vi "EX_REPORTS.vi"   [LabVIEW 2017]
uses:
  <vilib>/Utility/NIReport.llb/Append Report Text (str wrap).vi
  <vilib>/Utility/NIReport.llb/NI_report.lvclass
types:
  T1 = enum16{"maximized", "minimized", "normal", "no change"}
  T2 = cluster{"position (excel)":cluster{"row":i32, "column":i32}, "name (excel)":string, "bookmark (word)":string}
  T3 = enum16{"Standard Report", "HTML", "Word", "Excel"}
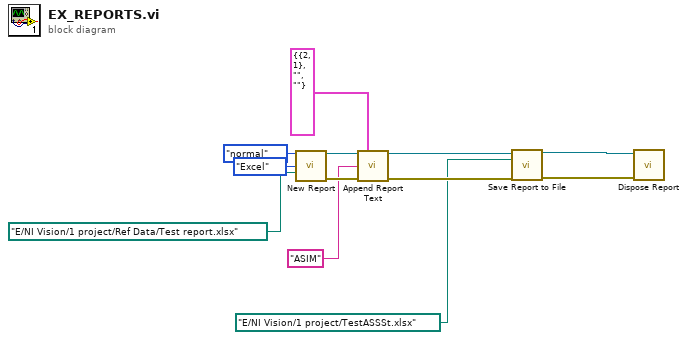
[diagram p0: block diagram]
diagram:
  n1 = call <vilib>:"New Report.vi"("window state (normal)"=T1."normal", "report type"=T3."Excel", "template (empty)"=path "E:/NI Vision/1 project/Ref Data/Test report.xlsx") -> ("report out"=w10:refnum<class "NI_report.lvclass">, "error out"=w9:errorcluster)  [unwired: 11 in]
  n2 = call-poly <vilib>:"Append Report Text.vi"("report in"=w10, "MS Office parameters"=T2 {"position (excel)"={"row"=2, "column"=1}, "name (excel)"="", "bookmark (word)"=""}, "text"="ASIM", "error in (no error)"=w9) -> ("report out"=w4:refnum<class "NI_report.lvclass">, "error out"=w6:errorcluster)  [unwired: 8 in, 2 out]
  n3 = call-dynamic "Save Report to File.vi"("report in"=w4, "report file path"=path "E:/NI Vision/1 project/TestASSSt.xlsx" ("template (empty)"), "error in (no error)"=w6) -> ("report out"=w3:refnum<class "NI_report.lvclass">, "error out"=w5:errorcluster)  [unwired: 11 in]
  n4 = call-dynamic "Dispose Report.vi"("report in"=w3, "error in (no error)"=w5) -> ()  [unwired: 13 in, 1 out]
